vi "tearDown.vi"(8 "error in (no error)":errorcluster, 11 "reference in":refnum<class "Deployment.lvclass">) -> (0 "error out":errorcluster, 3 "reference out":refnum<class "Deployment.lvclass">)   [LabVIEW 2020, in "Deployment.lvclass"]
doc: "tearDown runs after the test method has completed. Use this method to clean up any operations or references that were opened by setUp or the test method. Unit tests should be independent of other unit tests so this VI should ensure that the next test can run in a 'clean' test environment."
uses:
  Deployment.lvclass
  Deployment.lvclass/Deployment.ctl
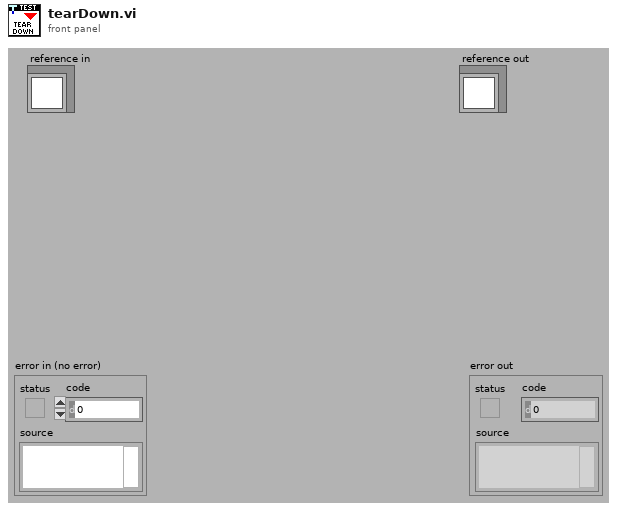
[diagram p1: front panel]
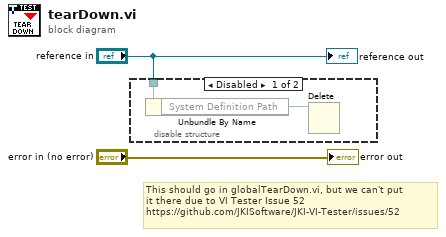
[diagram p0: block diagram]
diagram:
  # "This should go in globalTearDown.vi, but we can't put\nit there due to VI Tester Issue 52\nhttps://github.com/JKISoftware/JKI-VI-Tester/issues/52"
  n1 = disable-structure shown="Disabled" {
    disable-tunnel: "reference in" -> [w4 _]
    frame Disabled {
      n2 = Unbundle By Name(w4) -> ("System Definition Path"=w3:path)
      n3 = Delete(path (use dialog)=w3) -> ()  [unwired: 4 in, 3 out]
    }
    frame Enabled {
    }
  }
  "error out" <- "error in (no error)"
  "reference out" <- "reference in"
